vi "Channel Estimation Linear.vi"(11 "Ref":cdb[](array[numeric])) -> (0 "Numeric":dbl, 3 "Hest":cdb[](array[numeric]))   [LabVIEW 2014]
doc: "Estimates channel based on received refrence symbols and known refrecnce symbols"
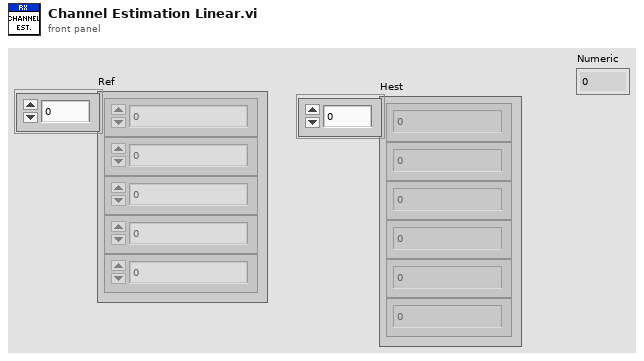
[diagram p1: front panel]
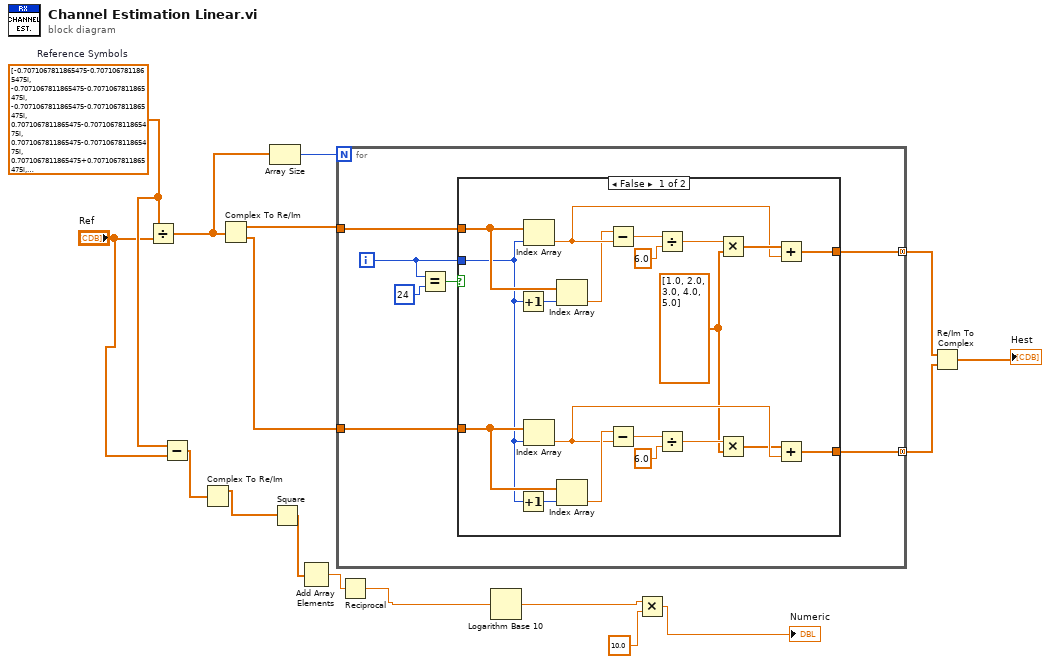
[diagram p0: block diagram]
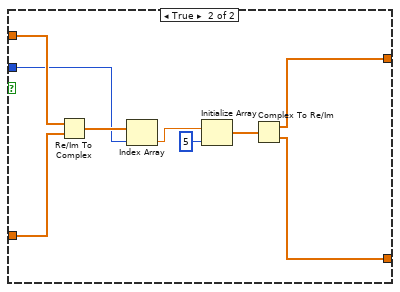
[diagram p2: hidden frame]
diagram:
  w10 = cdb[] [-0.7071067811865475-0.7071067811865475i, -0.7071067811865475-0.7071067811865475i, -0.7071067811865475-0.7071067811865475i, 0.7071067811865475-0.7071067811865475i, 0.7071067811865475-0.7071067811865475i, 0.7071067811865475+0.7071067811865475i, 0.7071067811865475-0.7071067811865475i, -0.7071067811865475-0.7071067811865475i, 0.7071067811865475+0.7071067811865475i, -0.7071067811865475+0.7071067811865475i, -0.7071067811865475-0.7071067811865475i, -0.7071067811865475+0.7071067811865475i, -0.7071067811865475+0.7071067811865475i, 0.7071067811865475-0.7071067811865475i, -0.7071067811865475+0.7071067811865475i, -0.7071067811865475+0.7071067811865475i, 0.7071067811865475-0.7071067811865475i, -0.7071067811865475+0.7071067811865475i, -0.7071067811865475-0.7071067811865475i, 0.7071067811865475-0.7071067811865475i, 0.7071067811865475+0.7071067811865475i, -0.7071067811865475-0.7071067811865475i, -0.7071067811865475-0.7071067811865475i, 0.7071067811865475-0.7071067811865475i, -0.7071067811865475-0.7071067811865475i, 0.7071067811865475-0.7071067811865475i, 0.7071067811865475-0.7071067811865475i, 0.7071067811865475+0.7071067811865475i, 0.7071067811865475+0.7071067811865475i, -0.7071067811865475-0.7071067811865475i, -0.7071067811865475+0.7071067811865475i, -0.7071067811865475+0.7071067811865475i, 0.7071067811865475-0.7071067811865475i, -0.7071067811865475-0.7071067811865475i, -0.7071067811865475+0.7071067811865475i, -0.7071067811865475-0.7071067811865475i, -0.7071067811865475+0.7071067811865475i, 0.7071067811865475-0.7071067811865475i, 0.7071067811865475+0.7071067811865475i, 0.7071067811865475+0.7071067811865475i, 0.7071067811865475-0.7071067811865475i, -0.7071067811865475-0.7071067811865475i, -0.7071067811865475+0.7071067811865475i, -0.7071067811865475+0.7071067811865475i, -0.7071067811865475-0.7071067811865475i, -0.7071067811865475-0.7071067811865475i, -0.7071067811865475+0.7071067811865475i, -0.7071067811865475+0.7071067811865475i, -0.7071067811865475+0.7071067811865475i, -0.7071067811865475+0.7071067811865475i]  # Reference Symbols
  n1 = Divide(x=w10, y="Ref") -> (x/y=w11:cdb[])
  n2 = Subtract(x=w10, y="Ref") -> (x-y=w8:cdb[])
  n3 = Complex To Re/Im(x + iy=w8) -> (x=w7:dbl[])  [unwired: 1 out]
  n4 = Complex To Re/Im(x + iy=w11) -> (x=w16:dbl[], y=w15:dbl[])
  n5 = Array Size(array=w11) -> (size(s)=w17:i32)
  n6 = Square(x=w7) -> (x^2=w3:dbl[])
  n7 = Add Array Elements(numeric array=w3) -> (sum=w2:dbl)
  n8 = for {
    N: w17 -> [_]
    tunnel: [w22] -> w13 mode=concatenating
    tunnel: w16 -> [w18]
    tunnel: w15 -> [w24]
    tunnel: [w21] -> w12 mode=concatenating
    i -> [w20]
    n9 = Equal?(x=w20, y=24) -> (x = y?=w19:bool)
    n10 = case shown="False" w19 {
      tunnel: w18 -> [w37 w53]
      tunnel: w24 -> [w29 w52]
      tunnel: [w27 w46] -> w22
      tunnel: [w26 w45] -> w21
      tunnel: w20 -> [w25 w50]
      frame False {
        w28 = dbl[] [1.0, 2.0, 3.0, 4.0, 5.0]
        n11 = Increment(x=w25) -> (x+1=w44:i32)
        n12 = Increment(x=w25) -> (x+1=w30:i32)
        n13 = Index Array(array=w37, index=w25) -> (element=w39:dbl)
        n14 = Index Array(array=w29, index=w25) -> (element=w35:dbl)
        n15 = Index Array(array=w37, index=w44) -> (element=w38:dbl)
        n16 = Index Array(array=w29, index=w30) -> (element=w36:dbl)
        n17 = Subtract(x=w38, y=w39) -> (x-y=w43:dbl)
        n18 = Subtract(x=w36, y=w35) -> (x-y=w31:dbl)
        n19 = Divide(x=w43, y=6.0) -> (x/y=w41:dbl)
        n20 = Divide(x=w31, y=6.0) -> (x/y=w33:dbl)
        n21 = Multiply(x=w41, y=w28) -> (x*y=w40:dbl[])
        n22 = Multiply(x=w33, y=w28) -> (x*y=w34:dbl[])
        n23 = Add(x=w40, y=w39) -> (x+y=w27:dbl[])
        n24 = Add(x=w34, y=w35) -> (x+y=w26:dbl[])
      }
      frame True {
        n25 = Re/Im To Complex(1:w52, 2:w53) -> (0:w51:cdb[])
        n26 = Index Array(array=w51, index=w50) -> (element=w49:cdb)
        n27 = Initialize Array(w49, 5 ("dimension size")) -> (w47:cdb[])
        n28 = Complex To Re/Im(x + iy=w47) -> (x=w46:dbl[], y=w45:dbl[])
      }
    }
  }
  n29 = Reciprocal(x=w2) -> (1/x=w1:dbl)
  n30 = Logarithm Base 10(1:w1) -> (0:w6:dbl)
  n31 = Multiply(x=w6, y=10.0) -> (x*y=→"Numeric":dbl)
  n32 = Re/Im To Complex(1:w12, 2:w13) -> (0:→"Hest":cdb[])
